vi "GetUnits.vi"(7 "Timeout (ms)":u32=2000, 8 "Error In":errorcluster, 11 "Sierra M100 In":refnum<visa-resource-name>) -> (0 "Error Out":errorcluster, 2 "Units":T1, 3 "Sierra M100 Out":refnum<visa-resource-name>)   [LabVIEW 2012, in "Sierra-M100.lvlib"]
doc: "This VI gets the units of measure for the flow rate. This includes the units for the setpoint and reading."
uses:
  Sierra-M100.lvlib
  Controls/Units.ctl
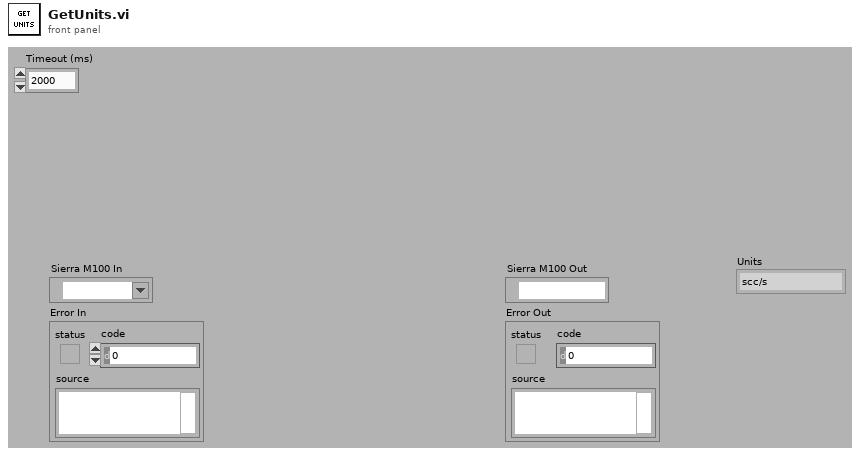
[diagram p1: front panel]
types:
  T1 = typedef "Sierra-M100.lvlib/Units.ctl" = enum16{"scc/s", "scc/m", "scc/H", "Ncc/s", "Ncc/m", "Ncc/H", "SCF/s", "SCF/m", "SCF/H", "NM3/s", "NM3/m", "NM3/H", "SM3/s", "SM3/m", "SM3/H", "sl/s", "sl/m", "sl/H", "NL/s", "NL/m", "Nl/H", "g/s", "g/m", "g/H", "kg/s", "kg/m", "kg/H", "lb/s", "lb/m", "lb/H"}
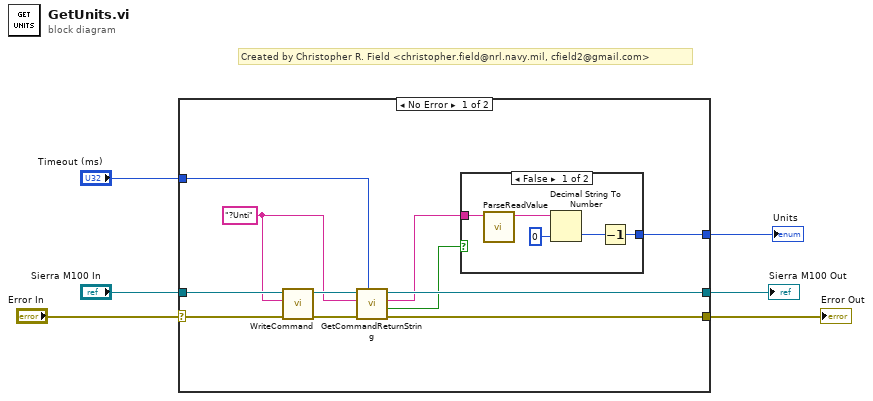
[diagram p0: block diagram]
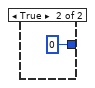
[diagram p2: hidden frame]
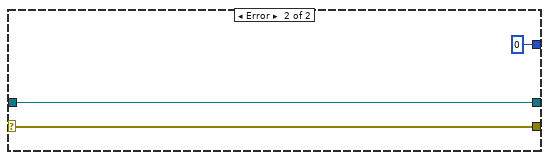
[diagram p3: hidden frame]
diagram:
  # "Created by Christopher R. Field <christopher.field@nrl.navy.mil, cfield2@gmail.com>"
  n1 = case shown="No Error" "Error In" {
    selector: "Error In" -> [w7 w25]
    tunnel: "Sierra M100 In" -> [w17 w26]
    tunnel: [w16 u16 0] -> w5
    tunnel: "Timeout (ms)" -> [w12 _]
    tunnel: [w11 w26] -> w3
    tunnel: [w10 w25] -> w2
    frame No Error {
      w13 = "?Unti"
      n2 = call "WriteCommand.vi"("Error In"=w7, "Command"=w13, "Smart Trak 2 In"=w17) -> ("Error Out"=w14:errorcluster, "Smart Trak 2 Out"=w15:refnum<visa-resource-name>)  [unwired: 5 in, 2 out]
      n3 = call "GetCommandReturnString.vi"("Timeout (ms)"=w12, "Error In"=w14, "Command"=w13, "Smart Trak 2 In"=w15) -> ("Error Out"=w10:errorcluster, "Timeout?"=w9:bool, "Return String"=w8:string, "Smart Trak 2 Out"=w11:refnum<visa-resource-name>)  [unwired: 4 in]
      n4 = case shown="False" w9 {
        tunnel: [w20 u16 0] -> w16
        tunnel: w8 -> [w18 _]
        frame False {
          n5 = call "ParseReadValue.vi"("Read Buffer"=w18) -> ("Value"=w19:string)  [unwired: 10 in]
          n6 = Decimal String To Number(string=w19, default (0L)=u16 0 ("default (0 I32)")) -> (number=w21:u16)  [unwired: 1 in, 1 out]
          n7 = Decrement(x=w21) -> (x-1=w20:u16)
        }
        frame True {
        }
      }
    }
    frame Error {
    }
  }
  "Sierra M100 Out" <- w3
  "Error Out" <- w2
  "Units" <- w5
